vi "Test Process Request Returns on Error.vi"(8 "error in (no error)":errorcluster, 11 "Process Test In":refnum<class "Process Test.lvclass">) -> (0 "error out":errorcluster, 3 "Process Test Out":refnum<class "Process Test.lvclass">)   [LabVIEW 2020, in "Process Test.lvclass"]
uses:
  Process Test.lvclass
  C:/Program Files (x86)/National Instruments/LabVIEW 2020/vi.lib/Asteme/LUnit/Test Case.lvclass
  Mock Process/Mock Process.lvclass
  C:/Users/anton/Documents/GitHub/Triarc-Framework/source/Framework/Process/Process.lvclass
  <vilib>/Asteme/LUnit/Test Case.lvclass/Test Case.ctl
  <vilib>/Asteme/LUnit/LUnit Assertion Result.lvclass/LUnit Assertion Result.ctl
  Framework/Process/Process.lvclass/Process.ctl
  <vilib>/Asteme/LUnit/Palette/Fail.vi
  <vilib>/Asteme/LUnit/Palette/Pass.vi
  <vilib>/Asteme/LUnit/Set Assertion Type.vi
  <vilib>/Asteme/LUnit/Variant to string.vi
  Framework/Process/Private/SubVIs/Wait for finish.vi
  Framework/Process/Protected/Messaging/Enqueue Message.vi
  Framework/Process/Private/SubVIs/Set Lifecycle State.vi
  Framework/Process/Public/Lifecycle/Get Lifecycle State.vi
  <vilib>/Asteme/LUnit/Add test result.vi
  <vilib>/Asteme/LUnit/LUnit Write Passed.vi
  <vilib>/Asteme/LUnit/LUnit Get Test Case.vi
  <vilib>/Asteme/LUnit/Assertion Result/LUnit Get Test Name.vi
  <vilib>/Asteme/LUnit/LUnit Write Message.vi
  <vilib>/Asteme/LUnit/LUnit Write Description.vi
  <vilib>/Asteme/LUnit/LUnit Write Assertion Type.vi
  <vilib>/Utility/error.llb/Clear Errors.vi
  <vilib>/Asteme/LUnit/Read Test Case Name.vi
  <vilib>/Utility/error.llb/Error Cluster From Error Code.vi
  <vilib>/Utility/Data Type/Get Type Information.vi
  <vilib>/Utility/LVClass/Get LV Class Name.vi
  <vilib>/ErrorRing/Error Ring.xnode
  <vilib>/Asteme/LUnit/LUnit Assertion Result.lvclass
  Framework/Process/Process.lvclass
  <vilib>/Asteme/LUnit/Test Case.lvclass
  C:/Users/anton/Documents/GitHub/Triarc-Framework/source/Framework Test/Base Class Test/Base Test.lvclass
  C:/Users/anton/Documents/GitHub/Triarc-Framework/source/Framework Test/Process Test/Process Test.lvclass
  C:/Users/anton/Documents/GitHub/Triarc-Framework/source/Framework/Base/Base.lvclass
  C:/Users/anton/Documents/GitHub/Triarc-Framework/source/Framework/Error Handler Interface/Error Handler Interface.lvclass
  C:/Users/anton/Documents/GitHub/Triarc-Framework/source/Framework/Logging/Logging.lvclass
  C:/Users/anton/Documents/GitHub/Triarc-Framework/source/Framework Test/Mock Process/Mock Process.lvclass
  C:/Users/anton/Documents/GitHub/Triarc-Framework/source/Framework/Helper Loop/Helper Loop.lvclass
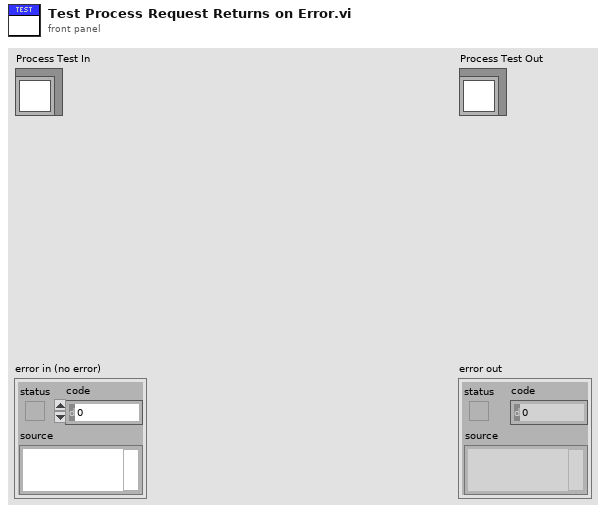
[diagram p1: front panel]
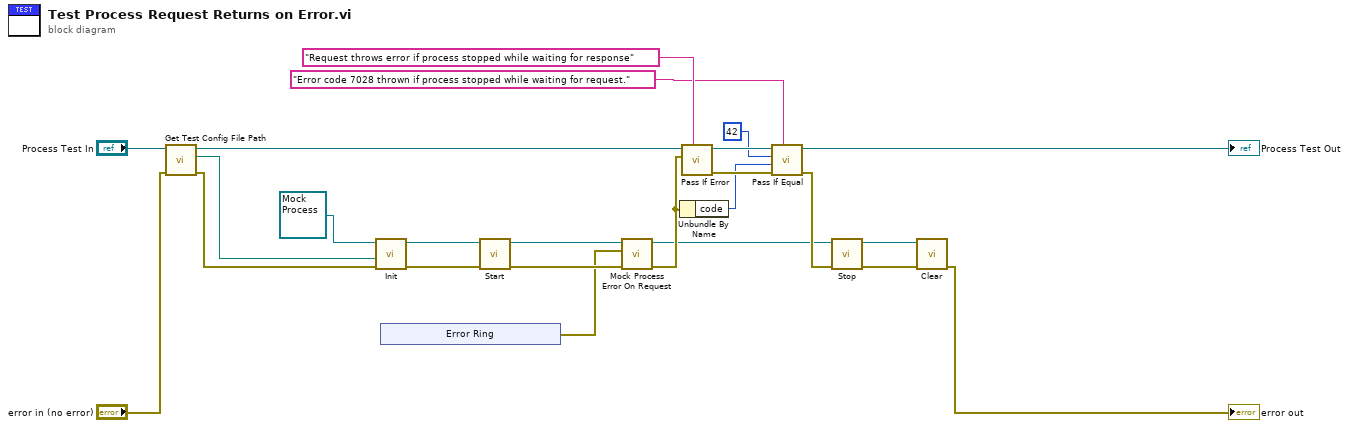
[diagram p0: block diagram]
diagram:
  n1 = call-dynamic "Get Test Config File Path.vi"("error in (no error)"="error in (no error)", "Base Class Test in"="Process Test In") -> ("error out"=w17:errorcluster, "Test config path"=w18:path, "Base Class Test out"=w20:refnum<class "Process Test.lvclass">)  [unwired: 7 in]
  n2 = call-dynamic "Init.vi"("error in (no error)"=w17, "Config File Path"=w18, "Mock Process In"=refnum<class "Mock Process.lvclass"> refnum ("Mock Process.lvclass")) -> ("error out"=w21:errorcluster, "Mock Process Out"=w22:refnum<class "Mock Process.lvclass">)  [unwired: 7 in]
  n3 = xnode "Error Ring"() -> ("error out"=w5:errorcluster)
  n4 = call "Start.vi"("error in (no error)"=w21, "Process In"=w22) -> ("error out"=w14:errorcluster, "Process Out"=w2:refnum<class "Mock Process.lvclass">)  [unwired: 8 in]
  n5 = call "Mock Process Error On Request.vi"("error in (no error)"=w14, "Mock Error"=w5, "Mock Process in"=w2) -> ("error out"=w9:errorcluster, "Mock Process out"=w1:refnum<class "Mock Process.lvclass">)  [unwired: 7 in]
  n6 = Unbundle By Name(w9) -> ("code"=w8:i32)
  n7 = call <vilib>:"Pass If Error.vi"("Description"="Request throws error if process stopped while waiting for response", "Assert error"=w9, "Test Case In"=w20) -> ("error out"=w10:errorcluster, "Test Case Out"=w13:refnum<class "Process Test.lvclass">)  [unwired: 7 in]
  n8 = call <vilib>:"Pass If Equal.vi"("Description"="Error code 7028 thrown if process stopped while waiting for request.", "error in (no error)"=w10, "Actual"=w8, "Expected"=42 ("code"), "Test Case In"=w13) -> ("error out"=w4:errorcluster, "Test Case Out"=→"Process Test Out":refnum<class "Process Test.lvclass">)  [unwired: 5 in]
  n9 = call "Stop.vi"("error in (no error)"=w4, "Process In"=w1) -> ("error out"=w3:errorcluster, "Process Out"=w24:refnum<class "Mock Process.lvclass">)  [unwired: 7 in, 1 out]
  n10 = call-dynamic "Clear.vi"("error in (no error)"=w3, "Mock Process In"=w24) -> ("error out"=→"error out":errorcluster)  [unwired: 9 in]
